vi "Create Frame.vi"(10 "color":u32(colorbox), 11 "frame":T1=enum."compact lib") -> (3 "frame picture":picture)   [LabVIEW 2017]
doc: "Creates icon frame."
uses:
  CTLs/Template Frame.ctl
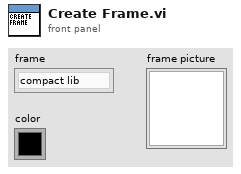
[diagram p1: front panel]
types:
  T1 = typedef "Template Frame.ctl" = enum16{"none", "compact lib"}
  T2 = cluster{"left":i16, "top":i16, "right":i16, "bottom":i16}
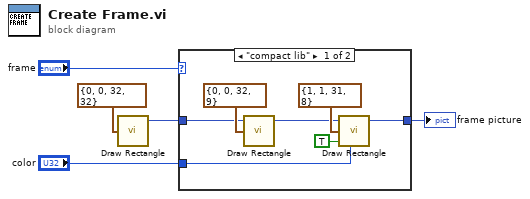
[diagram p0: block diagram]
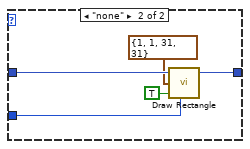
[diagram p2: hidden frame]
diagram:
  n1 = call <vilib>:"Draw Rectangle.vi"("rect"=T2 {"left"=0, "top"=0, "right"=32, "bottom"=32}) -> ("new picture"=w2:picture)  [unwired: 8 in]
  n2 = case shown="\"compact lib\"" "frame" {
    tunnel: w2 -> [w11 w17]
    tunnel: "color" -> [w8 w15]
    tunnel: [w6 w13] -> w5
    frame "compact lib" {
      n3 = call <vilib>:"Draw Rectangle.vi"("picture"=w11, "rect"=T2 {"left"=0, "top"=0, "right"=32, "bottom"=9}) -> ("new picture"=w9:picture)  [unwired: 7 in]
      n4 = call <vilib>:"Draw Rectangle.vi"("picture"=w9, "rect"=T2 {"left"=1, "top"=1, "right"=31, "bottom"=8}, "fill?(F)"=TRUE, "color(black)"=w8) -> ("new picture"=w6:picture)  [unwired: 5 in]
    }
    frame "none" {
      n5 = call <vilib>:"Draw Rectangle.vi"("picture"=w17, "rect"=T2 {"left"=1, "top"=1, "right"=31, "bottom"=31}, "fill?(F)"=TRUE, "color(black)"=w15) -> ("new picture"=w13:picture)  [unwired: 5 in]
    }
  }
  "frame picture" <- w5
